vi "vectornav data.vi"() -> ()   [LabVIEW 2010]
panel:
  in  "z-acceleration":dbl
  in  "y-acceleration":dbl
  in  "x-acceleration":dbl
  in  "z-magnetic":dbl
  in  "y-magnetic":dbl
  in  "x-magnetic":dbl
  in  "q[3]":dbl
  in  "q[2]":dbl
  in  "q[1]":dbl
  in  "q[0]":dbl
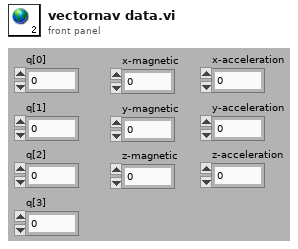
[diagram p1: front panel]
diagram:
